vi "Get Annotations For Parameter.vi"(10 "metadata value":T2(array[cluster]), 11 "parameter name":string) -> (3 "annotations":T1[](array[typedef]))   [LabVIEW 2020, in "MeasurementLink Measurement Server.lvlib"]
uses:
  MeasurementLink Measurement Server.lvlib
  TypeDefs/Parameter_AnnotationsEntry.ctl
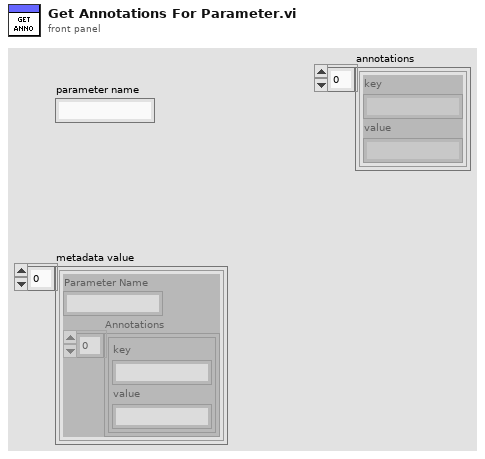
[diagram p1: front panel]
types:
  T1 = typedef "MeasurementLink Measurement Server.lvlib/Parameter_AnnotationsEntry.ctl" = cluster{"key":string, "value":string}
  T2 = cluster{"Parameter Name":string, "Annotations":T1[]}[]
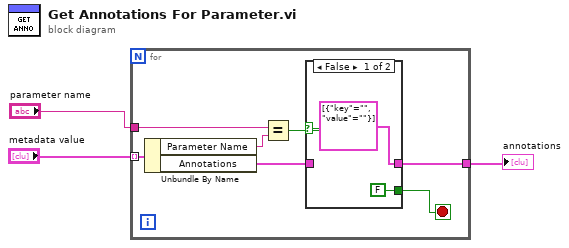
[diagram p0: block diagram]
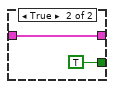
[diagram p2: hidden frame]
diagram:
  n1 = for {
    tunnel: "metadata value" -> [w9] mode=indexing
    tunnel: "parameter name" -> [w10]
    tunnel: [w4] -> w1
    stop <- w6 stop-if-true
    n2 = Unbundle By Name(w9) -> ("Parameter Name"=w8:string, "Annotations"=w5:T1[])
    n3 = Equal?(x=w10, y=w8) -> (x = y?=w7:bool)
    n4 = case shown="False" w7 {
      tunnel: [FALSE TRUE] -> w6
      tunnel: w5 -> [_ w13]
      tunnel: [T1[] [{"key"="", "value"=""}] ("Annotations") w13] -> w4
      frame False {
      }
      frame True {
      }
    }
  }
  "annotations" <- w1
